vi "SMS.vi"(0 "PhoneNumbers":string, 1 "SignName":string(combo)="斯坦道一体站", 5 "站点":string, 7 "时间标识":timestamp, 9 "内容":string, 11 "error in (no error)":errorcluster caption="错误输入（无错误）") -> (4 "headers":string caption="头部", 6 "body":string caption="体部", 15 "error out":errorcluster caption="错误输出")   [LabVIEW 2016]
uses:
  <vilib>/LVH/i3 JSON/JSON Generation/Create Value Files/Create Value - String.vi
  <vilib>/LVH/i3 OAuth/i3-oauth.lvlib
  <vilib>/httpClient/LabVIEWHTTPClient.lvlib
  <vilib>/LVH/i3 JSON/i3-json.lvlib
panel:
  out "长度":i32
  out "GET String":string
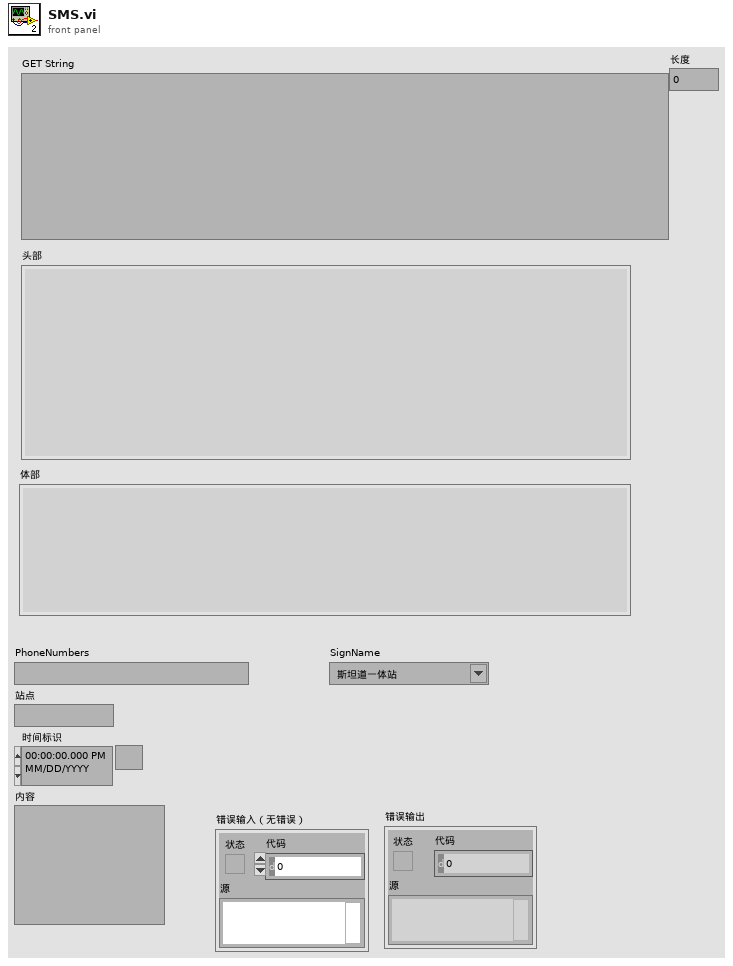
[diagram p1: front panel]
types:
  T1 = cluster{"Action":string, "Version":string, "RegionId":string, "PhoneNumbers":string, "SignName":string, "TemplateCode":string, "TemplateParam":string, "OutId":string}
  T2 = cluster{"AccessKeyId":string, "Timestamp":string, "Format":string, "SignatureMethod":string, "SignatureVersion":string, "SignatureNonce":string, "Signature":string}
  T3 = typedef "i3-oauth.lvlib/Name-Value Pair.ctl" = cluster{"Name":string, "Value":string}
  T4 = typedef "LabVIEWHTTPClient.lvlib/ClientHandle.ctl" = refnum<k1>
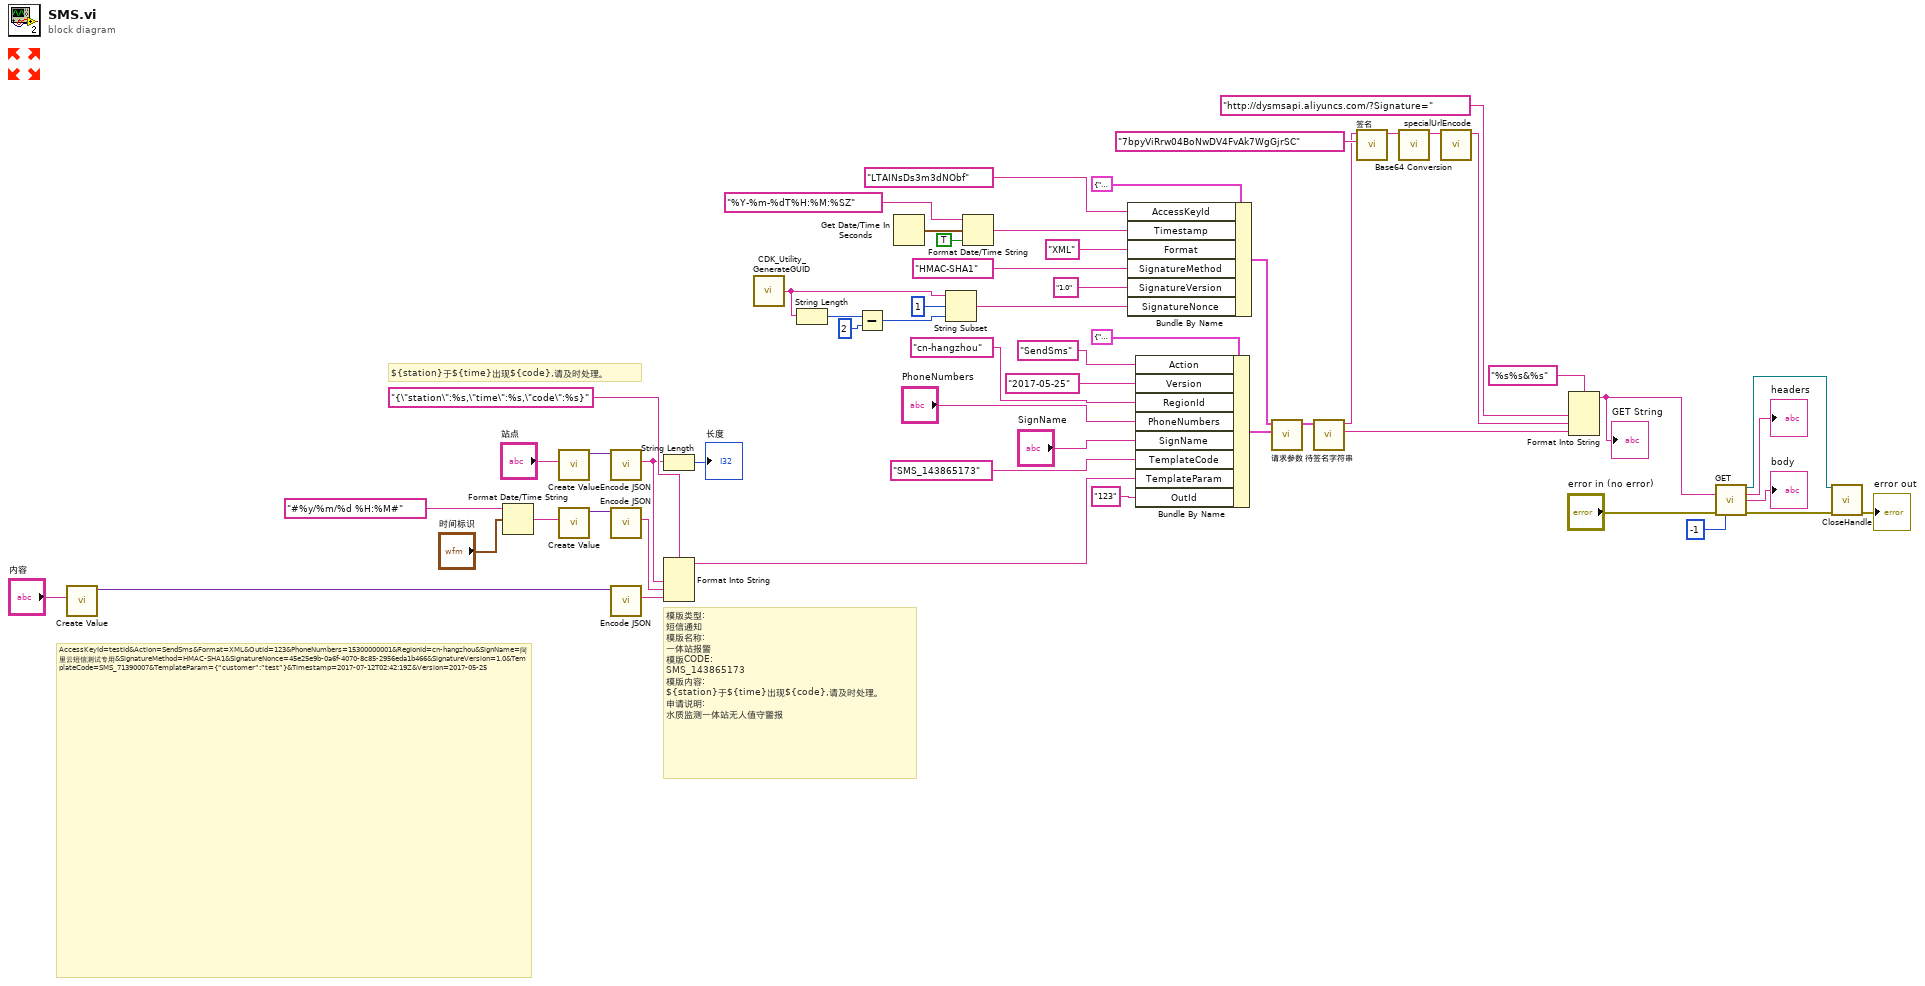
[diagram p0: block diagram]
diagram:
  # "模版类型:\n短信通知\n模版名称:\n一体站报警\n模版CODE:\nSMS_143865173\n模版内容:\n${station}于${time}出现${code},请及时处理。\n申请说明:\n水质监测一体站无人值守警报"
  # "${station}于${time}出现${code},请及时处理。"
  # "AccessKeyId=testId&Action=SendSms&Format=XML&OutId=123&PhoneNumbers=15300000001&RegionId=cn-hangzhou&SignName=阿里云短信测试专用&SignatureMethod=HMAC-SHA1&SignatureNonce=45e25e9b-0a6f-4070-8c85-2956eda1b466&SignatureVersion=1.0&TemplateCode=SMS_71390007&TemplateParam={“customer”:”test”}&Timestamp=2017-07-12T02:42:19Z&Version=2017-05-25"
  n1 = call-poly <vilib>:"Create Value.vi"("String"="内容") -> ("JSON Tree"=w3:variant)  [unwired: 9 in, 1 out]
  n2 = Format Date/Time String(time format string (%c)="#%y/%m/%d %H:%M#" ("时间格式字符串(%c)"), seconds (now)="时间标识") -> (date/time string=w5:string)  [unwired: 1 in]
  n3 = call-poly <vilib>:"Create Value.vi"("String"="站点") -> ("JSON Tree"=w17:variant)  [unwired: 9 in, 1 out]
  n4 = call-poly <vilib>:"Create Value.vi"("String"=w5) -> ("JSON Tree"=w6:variant)  [unwired: 9 in, 1 out]
  n5 = call <vilib>:"Encode JSON.vi"("JSON Tree"=w17) -> ("String"=w8:string)  [unwired: 5 in, 1 out]
  n6 = call <vilib>:"Encode JSON.vi"("JSON Tree"=w6) -> ("String"=w4:string)  [unwired: 5 in, 1 out]
  n7 = call <vilib>:"Encode JSON.vi"("JSON Tree"=w3) -> ("String"=w1:string)  [unwired: 5 in, 1 out]
  n8 = String Length(string=w8) -> (length=→"长度":i32)
  n9 = Format Into String(format string="{\"station\":%s,\"time\":%s,\"code\":%s}" ("TemplateParam"), w8, w4, w1) -> (resulting string=w15:string)  [unwired: 2 in, 1 out]
  n10 = call <resource>:"CDK_Utility_GenerateGUID.vi"() -> ("GUID"=w34:string)  [unwired: 9 in]
  n11 = String Length(string=w34) -> (length=w33:i32)
  n12 = Subtract(x=w33, y=2) -> (x-y=w31:i32)
  n13 = Get Date/Time In Seconds() -> (seconds since 1Jan1904=w29:timestamp)
  n14 = String Subset(string=w34, offset (0)=1 ("偏移量(0)"), length (rest)=w31) -> (substring=w30:string)
  n15 = Format Date/Time String(time format string (%c)="%Y-%m-%dT%H:%M:%SZ" ("时间格式字符串(%c)"), seconds (now)=w29, UTC format=TRUE ("UTC格式")) -> (date/time string=w26:string)
  n16 = Bundle By Name(cluster=T2 {"AccessKeyId"="", "Timestamp"="", "Format"="", "SignatureMethod"="", "SignatureVersion"="", "SignatureNonce"="", "Signature"=""} ("系统参数"), "AccessKeyId"="LTAINsDs3m3dNObf", "Timestamp"=w26, "Format"="XML", "SignatureMethod"="HMAC-SHA1", "SignatureVersion"="1.0", "SignatureNonce"=w30) -> (w48:T2)
  n17 = Bundle By Name(cluster=T1 {"Action"="", "Version"="", "RegionId"="", "PhoneNumbers"="", "SignName"="", "TemplateCode"="", "TemplateParam"="", "OutId"=""} ("业务参数"), "Action"="SendSms", "Version"="2017-05-25", "RegionId"="cn-hangzhou", "PhoneNumbers"="PhoneNumbers", "SignName"="SignName", "TemplateCode"="SMS_143865173", "TemplateParam"=w15, "OutId"="123") -> (w42:T1)
  n18 = call "请求参数.vi"("业务参数"=w42, "系统参数"=w48) -> ("已排序的数组"=w56:T3[])  [unwired: 9 in]
  n19 = call "待签名字符串.vi"("已排序的数组"=w56) -> ("sortQueryString"=w23:string, "StringToSign"=w39:string)  [unwired: 9 in]
  n20 = call "签名.vi"("consumer secret"="7bpyViRrw04BoNwDV4FvAk7WgGjrSC", "Signature Base string"=w39) -> ("Encoded Signature"=w54:string)  [unwired: 9 in]
  n21 = call <vilib>:"Base64 Conversion.vi"("String"=w54) -> ("Base64 String"=w36:string)  [unwired: 10 in]
  n22 = call "specialUrlEncode.vi"("str"=w36) -> ("UrlEncode"=w24:string)  [unwired: 10 in]
  n23 = Format Into String(format string="%s%s&%s" ("格式字符串"), "http://dysmsapi.aliyuncs.com/?Signature=" ("输入 1"), w24, w23) -> (resulting string=w25:string)  [unwired: 2 in, 1 out]
  "GET String" <- w25
  n24 = call <vilib>:"GET.vi"("url"=w25, "error in (no error)"="error in (no error)", "timeout (10000)"=-1) -> ("client handle out"=w20:T4, "headers"=→"headers":string, "body"=→"body":string, "error out"=w19:errorcluster)  [unwired: 9 in]
  n25 = call <vilib>:"CloseHandle.vi"("client handle"=w20, "error in (no error)"=w19) -> ("error out"=→"error out":errorcluster)  [unwired: 13 in]
